vi "_ViTree.vi"() -> ()   [LabVIEW 2017, in "TimerEngine.lvlib"]
uses:
  TimerEngine.lvlib
  TimerEngine.lvclass
panel:
  out "Timer Descriptions":string[](array[string])
  out "Timers":string[](array[string])
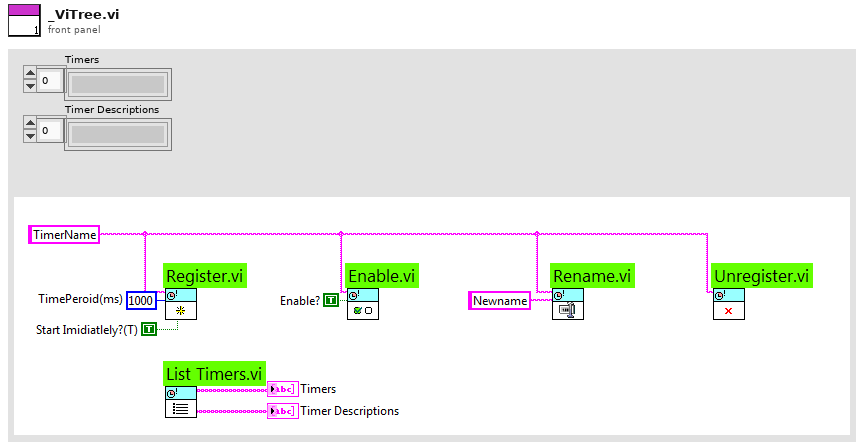
[diagram p1: front panel]
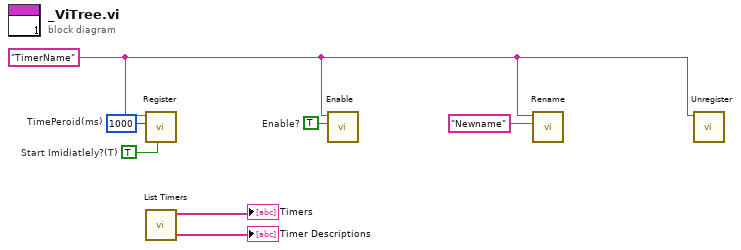
[diagram p0: block diagram]
diagram:
  w4 = TRUE  # Enable?
  w5 = TRUE  # Start Imidiatlely?(T)
  w6 = 1000  # TimePeroid(ms)
  w7 = "TimerName" ("Name")
  n1 = call "Register.vi"("Start Imidiatlely?(T)"=w5, "TimePeroid(ms)"=w6, "Name"=w7) -> ()  [unwired: 7 in, 2 out]
  n2 = call "List Timers.vi"() -> ("Timer Descriptions"=→"Timer Descriptions":string[], "Timers"=→"Timers":string[])  [unwired: 9 in, 1 out]
  n3 = call "Enable.vi"("Enable?"=w4, "Name"=w7) -> ()  [unwired: 9 in, 1 out]
  n4 = call "Rename.vi"("New Name"="Newname", "Name"=w7) -> ()  [unwired: 9 in, 1 out]
  n5 = call "Unregister.vi"("Name"=w7) -> ()  [unwired: 10 in, 1 out]
